vi "Day 10.2 - Complete sequence.vi"(11 "input":string[](array[string])) -> (3 "output":u64)   [LabVIEW 2021]
uses:
  0728f00d-960a-4c61-b2ef-1b64b89bb78b.vi
  <vilib>/Comparison/Less/Less Functor/Less Functor.lvclass
panel:
  out "Scores":u64[](array[numeric])
  out "Mismatched close":string[](array[string])
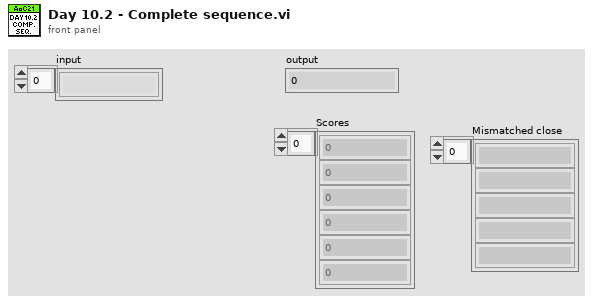
[diagram p1: front panel]
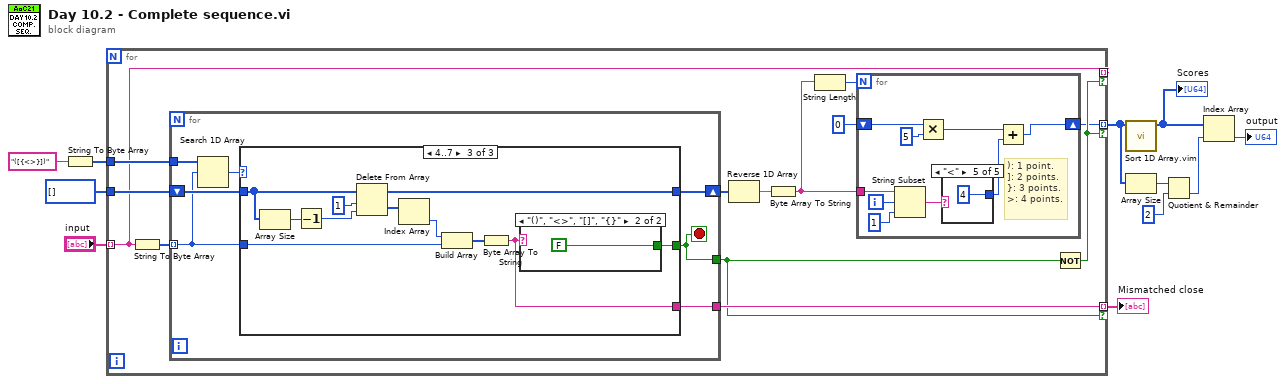
[diagram p0: block diagram]
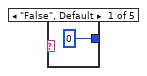
[diagram p2: hidden frame]
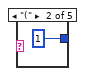
[diagram p3: hidden frame]
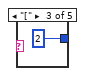
[diagram p4: hidden frame]
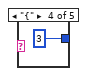
[diagram p5: hidden frame]
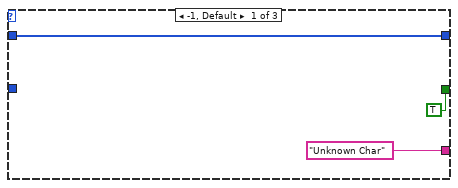
[diagram p6: hidden frame]
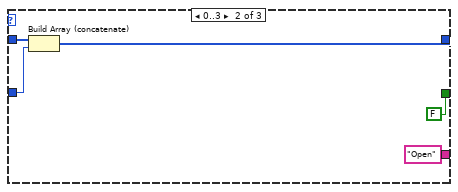
[diagram p7: hidden frame]
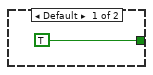
[diagram p8: hidden frame]
diagram:
  n1 = String To Byte Array(string="([{<>}])" ("regular expression")) -> (unsigned byte array=w8:u8[])
  n2 = for {
    tunnel: "input" -> [w20] mode=indexing
    tunnel: i32[] [] -> [w24]
    tunnel: w8 -> [w23]
    tunnel: [w21] -> w7 mode=indexing if=w19
    tunnel: [w20] -> _ mode=indexing if=w18
    tunnel: [w12] -> w3 mode=indexing if=w18
    n3 = String To Byte Array(string=w20) -> (unsigned byte array=w22:u8[])
    n4 = for {
      shift-right: [w42] -> w13
      shift-left: w24 -> [w43]
      tunnel: w23 -> [w45]
      tunnel: w22 -> [w41] mode=indexing
      tunnel: [w40] -> w21
      tunnel: [w39] -> w19
      stop <- w39 stop-if-true
      n5 = Search 1D Array(1D array=w45, element=w41) -> (index of element=w44:i32)  [unwired: 1 in]
      n6 = case shown="4..7" w44 {
        tunnel: [w48 w51 w60] -> w42
        tunnel: w43 -> [w48 w53 w61]
        tunnel: w41 -> [_ w52 w57]
        tunnel: [TRUE FALSE w54] -> w39
        tunnel: ["Unknown Char" ("string") "Open" ("string") w55] -> w40
        frame -1, Default {
        }
        frame 0..3 {
          n7 = Build Array (concatenate)(w53, w52) -> (w51:i32[])
        }
        frame 4..7 {
          n8 = Array Size(array=w61) -> (size(s)=w64:i32)
          n9 = Decrement(x=w64) -> (x-1=w63:i32)
          n10 = Delete From Array(array=w61, length=1, index=w63) -> (deleted portion=w59:i32[], array with subset deleted=w60:i32[])
          n11 = Index Array(array=w59) -> (element=w58:i32)  [unwired: 1 in]
          n12 = Build Array(w58, w57) -> (w56:i32[])
          n13 = Byte Array To String(unsigned byte array=w56) -> (string=w55:string)
          n14 = case shown="\"()\", \"<>\", \"[]\", \"{}\"" w55 {
            tunnel: [TRUE FALSE] -> w54
            frame Default {
            }
            frame "()", "<>", "[]", "{}" {
            }
          }
        }
      }
    }
    n15 = Reverse 1D Array(array=w13) -> (reversed array=w17:i32[])
    n16 = Byte Array To String(unsigned byte array=w17) -> (string=w15:string)
    n17 = String Length(string=w15) -> (length=w16:i32)
    n18 = for {
      N: w16 -> [_]
      tunnel: w15 -> [w31]
      shift-right: [w26] -> w12
      shift-left: u64 0 -> [w30]
      i -> [w25]
      # "): 1 point.\n]: 2 points.\n}: 3 points.\n>: 4 points."
      n19 = String Subset(string=w31, offset (0)=w25, length (rest)=1 ("offset (0)")) -> (substring=w32:string)
      n20 = Multiply(x=w30, y=u64 5) -> (x*y=w28:u64)
      n21 = case shown="\"<\"" w32 {
        tunnel: [0 1 2 3 4] -> w27
        frame "False", Default {
        }
        frame "(" {
        }
        frame "[" {
        }
        frame "{" {
        }
        frame "<" {
        }
      }
      n22 = Add(x=w28, y=w27) -> (x+y=w26:u64)
    }
    n23 = Not(x=w19) -> (.not. x?=w18:bool)
  }
  "Mismatched close" <- w7
  n24 = call "Sort 1D Array.vim"("unsorted array"=w3) -> ("sorted array"=w2:u64[])  [unwired: 10 in]
  "Scores" <- w2
  n25 = Array Size(array=w3) -> (size(s)=w6:i32)
  n26 = Quotient & Remainder(x=w6, y=2) -> (floor(x/y)=w4:i32)  [unwired: 1 out]
  n27 = Index Array(array=w2, index=w4) -> (element=→"output":u64)
